vi "ziGetEventDemodVector.vi"(8 "Error In":errorcluster, 11 "Handle In":T2 {"Handle" format="0x%08x"; "Conn" format="0x%08x"}) -> (0 "Error Out":errorcluster, 2 "Demod Vector Out":T1, 3 "Handle Out":T2 {"Handle" format="0x%08x"; "Conn" format="0x%08x"})   [LabVIEW 2009, in "Zurich Instruments LabOne.lvlib"]
uses:
  <instrlib>/Zurich Instruments LabOne/Zurich Instruments LabOne.lvlib
  <instrlib>/Zurich Instruments LabOne/Public/ziTypeHandle.ctl
  <instrlib>/Zurich Instruments LabOne/Public/Data/ziTypeDemodVectorEx.ctl
  <instrlib>/Zurich Instruments LabOne/Private/ziLV32.dll
panel:
  in  "Demod Vector In":T1
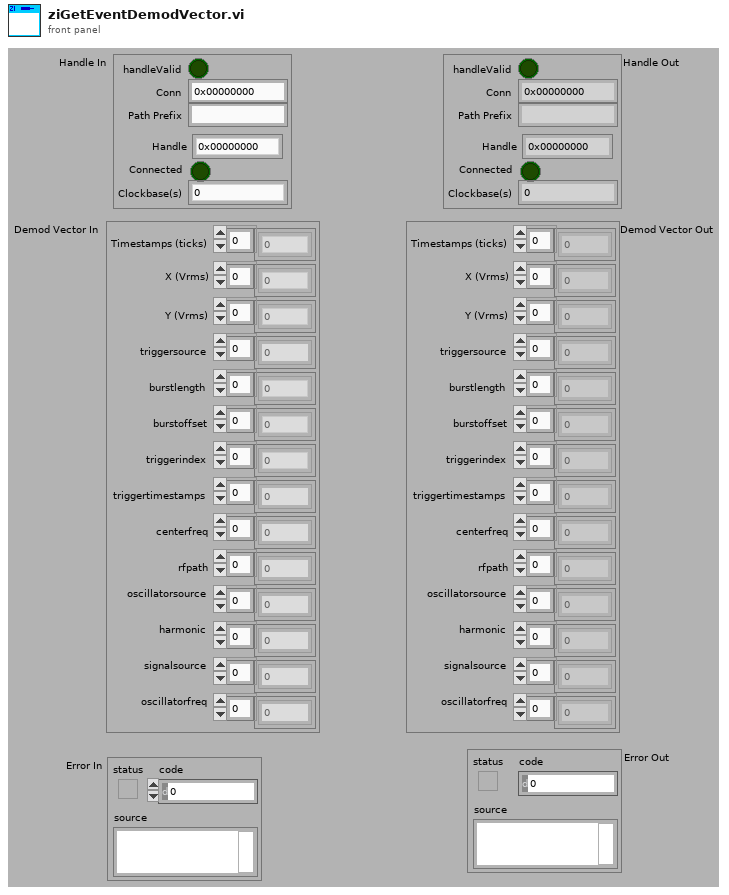
[diagram p1: front panel]
types:
  T1 = typedef "Zurich Instruments LabOne.lvlib/ziTypeDemodVectorEx.ctl" = cluster{"Timestamps (ticks)":u64[], "X (Vrms)":dbl[], "Y (Vrms)":dbl[], "triggersource":u8[], "burstlength":u32[], "burstoffset":u32[], "triggerindex":u32[], "triggertimestamps":u64[], "centerfreq":dbl[], "rfpath":u8[], "oscillatorsource":u16[], "harmonic":u16[], "signalsource":u16[], "oscillatorfreq":dbl[]}
  T2 = typedef "Zurich Instruments LabOne.lvlib/ziTypeHandle.ctl" = cluster{"handleValid":bool, "Conn":u64, "Path Prefix":string, "Handle":u64, "Connected":bool, "Clockbase(s)":dbl}
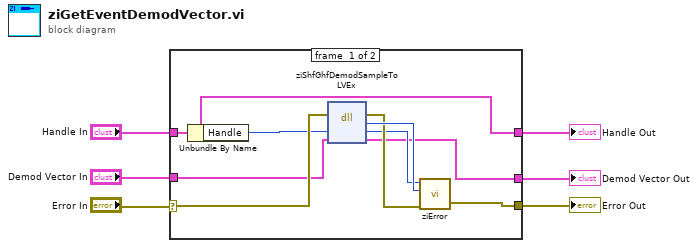
[diagram p0: block diagram]
diagram:
  n1 = case shown="No Error" "Error In" {
    selector: "Error In" -> [w14 w17]
    tunnel: "Handle In" -> [w10 w18]
    tunnel: [w10 w18] -> w5
    tunnel: [w15 w17] -> w4
    tunnel: [w8 w16] -> w2
    tunnel: "Demod Vector In" -> [w7 w16]
    frame #0 {
      n2 = Unbundle By Name(w10) -> ("Handle"=w13:u64)
      n3 = dll-call lib="C:/Program Files (x86)/National Instruments/LabVIEW 2009/instr.lib/Zurich Instruments LabOne/Private/ziLV*.*" fn="ziShfGhfDemodSampleToLVEx"(error in=w14, "ziEventBuffer"=w13, w7) -> (error out=w11:errorcluster, "return type"=w12:u32, "ziEventBuffer"=w9:u64, w8:T1)  [unwired: 2 in, 1 out]
      n4 = call <instrlib>:"ziError.vi"("Conn"=w9, "ziErrorCode"=w12, "Error In"=w11) -> ("Error Out"=w15:errorcluster)  [unwired: 2 in, 1 out]
    }
    frame #1 {
    }
  }
  "Handle Out" <- w5
  "Error Out" <- w4
  "Demod Vector Out" <- w2
